vi "subVIwithState.vi"(1 "u":dbl) -> (0 "y":dbl[](array[numeric]) format="%.4f")   [LabVIEW 2023]
uses:
  <vilib>/Analysis/baseanly.llb/A x Vector.vi
  <vilib>/Analysis/NI_AALBase.lvlib
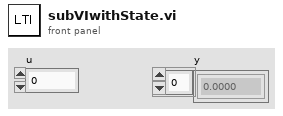
[diagram p1: front panel]
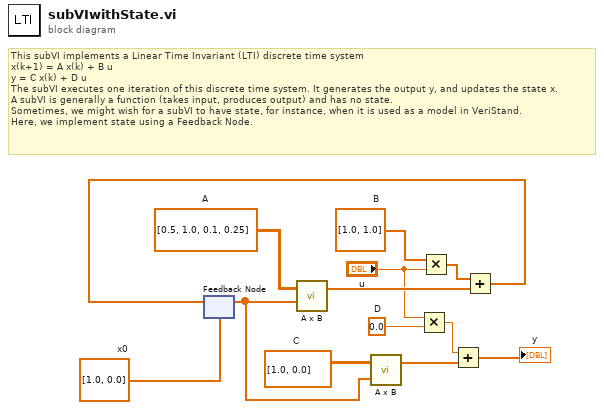
[diagram p0: block diagram]
diagram:
  w3 = 0.0  # D
  w6 = dbl[][] [[1.0, 0.0]]  # C
  w11 = dbl[] [1.0, 1.0]  # B
  w12 = dbl[][] [[0.5, 1.0], [0.1, 0.25]]  # A
  w13 = dbl[] [1.0, 0.0]  # x0
  # "This subVI implements a Linear Time Invariant (LTI) discrete time system\nx(k+1) = A x(k) + B u\ny = C x(k) + D u\nThe subVI executes one iteration of this discrete time system. It generates the output y, and updates the state x.\nA subVI is generally a function (takes input, produces output) and has no state.\nSometimes, we might wish for a subVI to have state, for instance, when it is used as a model in VeriStand.\nHere, we implement state using a Feedback Node."
  n1 = feedback #1(w13) -> (w7:dbl[])
  n2 = call-poly <vilib>:"A x B.vi"("Vector"=w7, "A"=w12) -> ("A x Vector"=w9:dbl[])  [unwired: 1 out]
  n3 = call-poly <vilib>:"A x B.vi"("Vector"=w7, "A"=w6) -> ("A x Vector"=w5:dbl[])  [unwired: 1 out]
  n4 = Multiply(x="u", y=w3) -> (x*y=w4:dbl)
  n5 = Multiply(x=w11, y="u") -> (x*y=w10:dbl[])
  n6 = Add(x=w4, y=w5) -> (x+y=→"y":dbl[])
  n7 = Add(x=w10, y=w9) -> (x+y=w8:dbl[])
  n8 = feedback-in #1(w8) -> ()
